vi "Execute.vi"(8 "error in (no error)":errorcluster, 9 "System in":refnum<class "System.lvclass">, 10 "Command in":refnum<class "Command.lvclass">, 11 "DM-MaintainPower-State in":refnum<class "DM-MaintainPower-State.lvclass">) -> (0 "error out":errorcluster, 2 "Next State":refnum<class "State.lvclass">, 3 "DM-MaintainPower-State out":refnum<class "DM-MaintainPower-State.lvclass">)   [LabVIEW 2013, in "DM-MaintainPower-State.lvclass"]
uses:
  DM-MaintainPower-State.lvclass
  Commands/Command/Command.lvclass
  Systems/System/System.lvclass
  State/State.lvclass
  Systems/DriveMotors/DriveMotors.lvclass
  Commands/DM-SetPower-Command/DM-SetPower-Command.lvclass
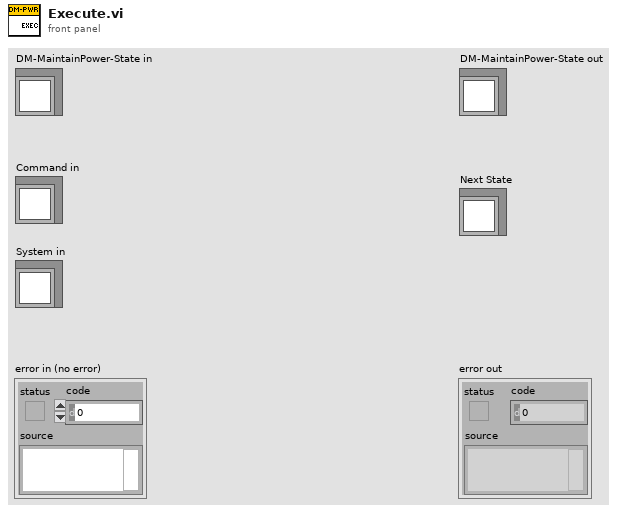
[diagram p1: front panel]
types:
  T1 = typedef "DM-SetPower-Command.lvclass/DM-SetPower-Command-Arguments.ctl" = cluster{"Power":dbl}
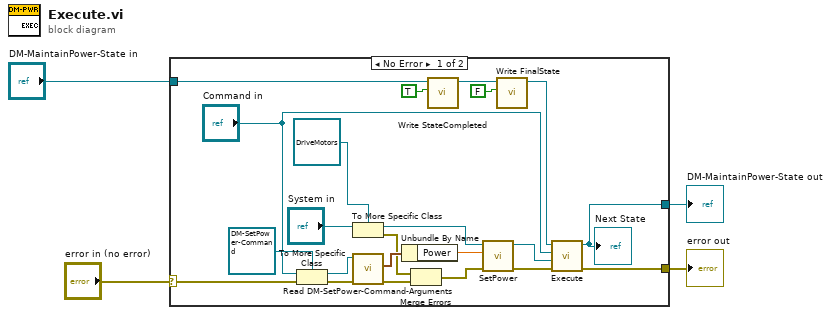
[diagram p0: block diagram]
diagram:
  n1 = case shown="No Error" "error in (no error)" {
    selector: "error in (no error)" -> [w9 w27]
    tunnel: [w26 w27] -> w3
    tunnel: "DM-MaintainPower-State in" -> [w14 w28]
    tunnel: [w17 w28] -> w1
    frame No Error {
      n2 = To More Specific Class(target class=refnum<class "DM-SetPower-Command.lvclass"> refnum ("DM-SetPower-Command.lvclass"), reference="Command in", error in=w9) -> (specific class reference=w22:refnum<class "DM-SetPower-Command.lvclass">, error out=w8:errorcluster)
      n3 = To More Specific Class(target class=refnum<class "DriveMotors.lvclass"> refnum ("DriveMotors in"), reference="System in") -> (specific class reference=w10:refnum<class "DriveMotors.lvclass">, error out=w7:errorcluster)  [unwired: 1 in]
      n4 = call-dynamic "Read DM-SetPower-Command-Arguments.vi"("error in (no error)"=w8, "DM-SetPower-Command in"=w22) -> ("error out"=w6:errorcluster, "DM-SetPower-Command-In"=w21:T1)  [unwired: 7 in, 1 out]
      n5 = Unbundle By Name(w21) -> ("Power"=w20:dbl)
      n6 = Merge Errors(w7, w6) -> (w5:errorcluster)
      n7 = call-dynamic "Write StateCompleted.vi"("StateCompleted"=TRUE, "State in"=w14) -> ("State out"=w15:refnum<class "DM-MaintainPower-State.lvclass">)  [unwired: 8 in, 1 out]
      n8 = call-dynamic "SetPower.vi"("error in (no error)"=w5, "MotorPower"=w20, "DriveMotors in"=w10) -> ("error out"=w16:errorcluster, "DriveMotors out"=w18:refnum<class "DriveMotors.lvclass">)  [unwired: 7 in]
      n9 = call-dynamic "Write FinalState.vi"("FinalState"=FALSE, "State in"=w15) -> ("State out"=w13:refnum<class "DM-MaintainPower-State.lvclass">)  [unwired: 8 in, 1 out]
      n10 = call-parent "Execute.vi"("error in (no error)"=w16, "System in"=w18, "Command in"="Command in", "State in"=w13) -> ("error out"=w26:errorcluster, "State out"=w17:refnum<class "DM-MaintainPower-State.lvclass">)  [unwired: 5 in, 1 out]
      "Next State" <- w17
    }
    frame Error {
    }
  }
  "error out" <- w3
  "DM-MaintainPower-State out" <- w1
